vi "Filter to applicable styles.vi"(8 "Error in":errorcluster, 10 "Selectors":string[](array[string]), 11 "LSS styles":T1[](array[typedef])) -> (0 "Error out":errorcluster, 3 "Applicable styles":T1[](array[typedef]))   [LabVIEW 2019, in "LSS.lvlib"]
doc: "For a given set of selectors, return the set of Style Sheet properties that should be applied to the control whose selectors are being analyzed.\n\n<b>Inputs:</b>\n<b>LSS Styles</b> - List of all LSS styles that are in memory.\n<b>Selectors</b> - This VI sorts through this list of selectors to find which LSS styles apply.\n<b>Error In</b> - Standard Error In terminal.\n\n<b>Outputs:</b>\n<b>Applicable styles</b> - List of applicable styles for the selectors input.\n<b>Error Out</b> - Standard Error Out terminal."
uses:
  LSS.lvlib
  Controls/Style.ctl
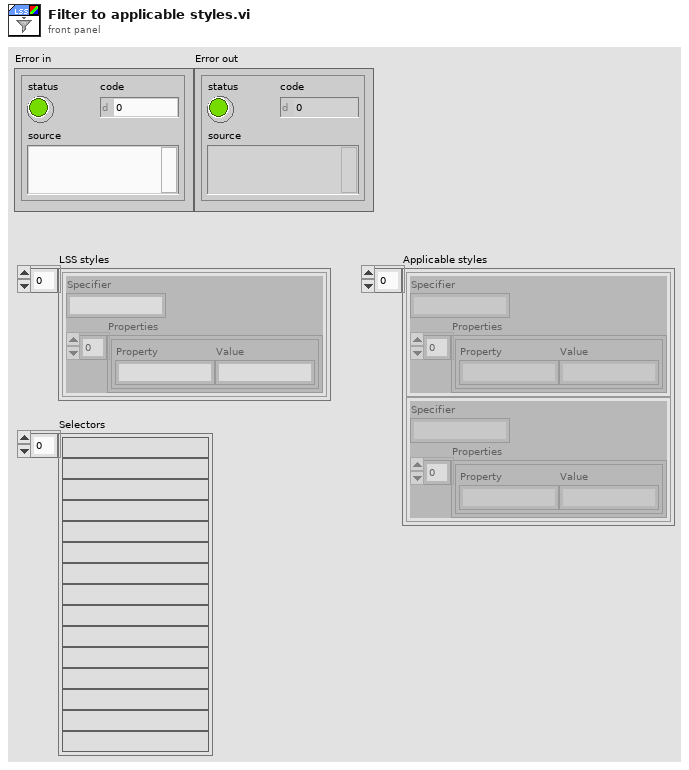
[diagram p1: front panel]
types:
  T1 = typedef "LSS.lvlib/Style.ctl" = cluster{"Specifier":string, "Properties":cluster{"Property":string, "Value":string}[]}
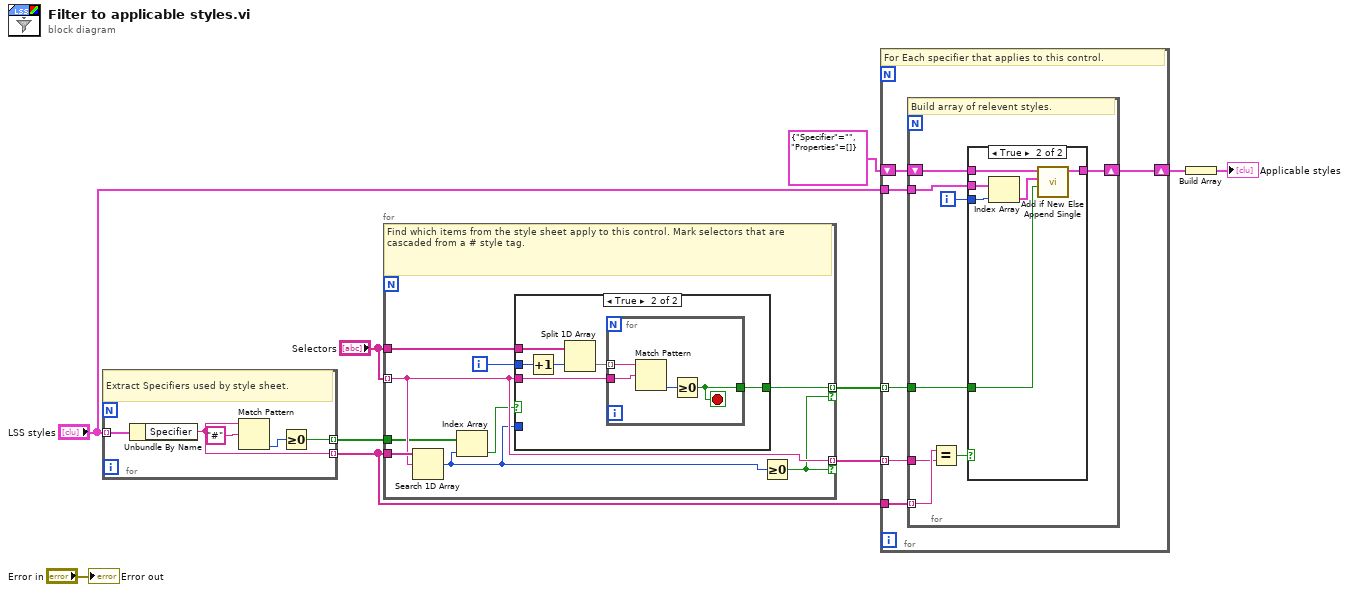
[diagram p0: block diagram]
diagram:
  n1 = for {
    tunnel: "LSS styles" -> [w15] mode=indexing
    tunnel: [w14] -> w3 mode=indexing
    tunnel: [w11] -> w6 mode=indexing
    # "Extract Specifiers used by style sheet."
    n2 = Unbundle By Name(w15) -> ("Specifier"=w14:string)
    n3 = Match Pattern(string=w14, regular expression="#") -> (offset past match=w12:i32)  [unwired: 1 in, 3 out]
    n4 = Greater Or Equal To 0?(x=w12) -> (x >= 0?=w11:bool)
  }
  n5 = for {
    tunnel: "Selectors" -> [w23] mode=indexing
    tunnel: w3 -> [w24]
    tunnel: [w23] -> w2 mode=indexing if=w21
    tunnel: w6 -> [w20]
    tunnel: [w22] -> w1 mode=indexing if=w21
    tunnel: "Selectors" -> [w16]
    i -> [w17]
    # "Find which items from the style sheet apply to this control. Mark selectors that are cascaded from a # style tag."
    n6 = Search 1D Array(1D array=w24, element=w23) -> (index of element=w19:i32)  [unwired: 1 in]
    n7 = Index Array(array=w20, index=w19) -> (element=w18:bool)
    n8 = case shown="True" w18 {
      tunnel: w23 -> [_ w30]
      tunnel: w19 -> [_ _]
      tunnel: [_ w26] -> w22
      tunnel: w17 -> [_ w28]
      tunnel: w16 -> [_ w29]
      frame False {
      }
      frame True {
        n9 = Increment(x=w28) -> (x+1=w25:i32)
        n10 = Split 1D Array(array=w29, index=w25) -> (second subarray=w27:string[])  [unwired: 1 out]
        n11 = for {
          tunnel: w27 -> [w34] mode=indexing
          tunnel: w30 -> [w33]
          tunnel: [w31] -> w26
          stop <- w31 stop-if-true
          n12 = Match Pattern(string=w34, regular expression=w33) -> (offset past match=w32:i32)  [unwired: 1 in, 3 out]
          n13 = Greater Or Equal To 0?(x=w32) -> (x >= 0?=w31:bool)
        }
      }
    }
    n14 = Greater Or Equal To 0?(x=w19) -> (x >= 0?=w21:bool)
  }
  n15 = for {
    tunnel: w2 -> [w36] mode=indexing
    tunnel: w3 -> [w37]
    tunnel: "LSS styles" -> [w40]
    shift-right: [w38] -> w10
    shift-left: T1 {"Specifier"="", "Properties"=[]} -> [w39]
    tunnel: w1 -> [w35] mode=indexing
    # "For Each specifier that applies to this control."
    n16 = for {
      tunnel: w40 -> [w48]
      shift-right: [w46] -> w38
      shift-left: w39 -> [w47]
      tunnel: w37 -> [w45] mode=indexing
      tunnel: w36 -> [w44]
      tunnel: w35 -> [w41]
      i -> [w43]
      # "Build array of relevent styles."
      n17 = Equal?(x=w45, y=w44) -> (x = y?=w42:bool)
      n18 = case shown="True" w42 {
        tunnel: w48 -> [_ w55]
        tunnel: w47 -> [w49 w53]
        tunnel: [w49 w51] -> w46
        tunnel: w43 -> [_ w54]
        tunnel: w41 -> [_ w50]
        frame False {
        }
        frame True {
          n19 = Index Array(array=w55, index=w54) -> (element=w52:T1)
          n20 = call "Add if New Else Append Single.vi"("Cascaded Static Value"=w50, "New Element"=w52, "Style In"=w53) -> ("Style Out"=w51:T1)  [unwired: 8 in]
        }
      }
    }
  }
  n21 = Build Array(w10) -> (→"Applicable styles":T1[])
  "Error out" <- "Error in"
